vi "calc T.vi"(7 "DAQ state cluster in in":T1 {"T cont"."utility"."therm volt" format="%_6g"; "T cont"."T status"."Temp" format="%_6g"}) -> (8 "DAQ state cluster out":T1 {"T cont"."utility"."therm volt" format="%_6g"; "T cont"."T status"."Temp" format="%_6g"})   [LabVIEW 2019]
doc: "This subVI is a component of the meas T state of the DAQ state machine in the thermistor experiment.\n\nThis subVI calculates the current time and the thermistor temperature from the raw voltage measurement.\n\nPaul K Dixon\nP3600\nCSUSB Physics"
uses:
  typedefs/DAQ T state cluster.ctl
  typedefs/DAQ T state enum.ctl
  typedefs/temp cont cluster.ctl
  typedefs/temp exec cluster.ctl
  typedefs/temp mode enum.ctl
  typedefs/temp indicator.ctl
  typedefs/temp cont utility.ctl
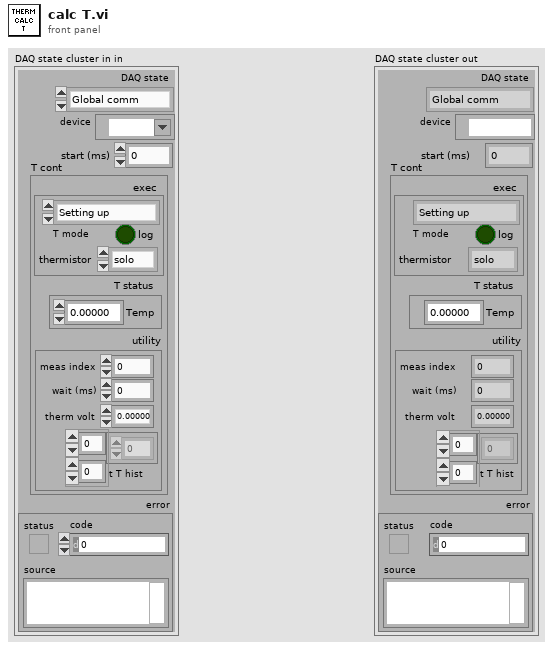
[diagram p1: front panel]
types:
  T1 = typedef "DAQ T state cluster.ctl" = cluster{"DAQ state":T2, "device":tag, "start (ms)":i32, "error":errorcluster, "T cont":T3}
  T2 = typedef "DAQ T state enum.ctl" = enum16{"Global comm", "Meas T ", "Wait", "Exit"}
  T3 = typedef "temp cont cluster.ctl" = cluster{"exec":T4, "T status":T6, "utility":T7}
  T4 = typedef "temp exec cluster.ctl" = cluster{"T mode":T5, "log":bool, "thermistor":enum16{"solo", "bug"}}
  T5 = typedef "temp mode enum.ctl" = enum16{"Setting up", "Listening to exec", "Exit"}
  T6 = typedef "temp indicator.ctl" = cluster{"Temp":dbl}
  T7 = typedef "temp cont utility.ctl" = cluster{"meas index":i32, "wait (ms)":i32, "therm volt":dbl, "t T hist":dbl[][]}
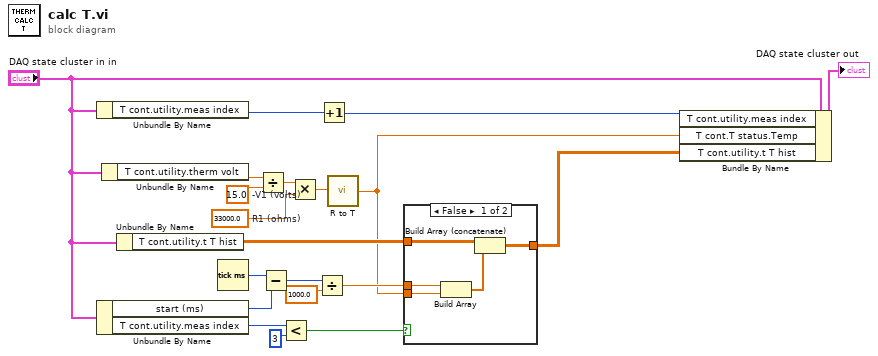
[diagram p0: block diagram]
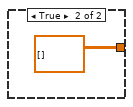
[diagram p2: hidden frame]
diagram:
  w18 = 15.0  # -V1 (volts)
  w16 = 33000.0  # R1 (ohms)
  n1 = Unbundle By Name("DAQ state cluster in in") -> ("T cont.utility.meas index"=w6:i32)
  n2 = Unbundle By Name("DAQ state cluster in in") -> ("start (ms)"=w12:i32, "T cont.utility.meas index"=w4:i32)
  n3 = Unbundle By Name("DAQ state cluster in in") -> ("T cont.utility.therm volt"=w19:dbl)
  n4 = Unbundle By Name("DAQ state cluster in in") -> ("T cont.utility.t T hist"=w14:dbl[][])
  n5 = Tick Count (ms)() -> (millisecond timer value=w13:u32)
  n6 = Divide(x=w19, y=w18) -> (x/y=w17:dbl)
  n7 = Subtract(x=w13, y=w12) -> (x-y=w11:u32)
  n8 = Less?(x=w4, y=3) -> (x < y?=w2:bool)
  n9 = Multiply(x=w17, y=w16) -> (x*y=w15:dbl)
  n10 = Divide(x=w11, y=1000.0) -> (x/y=w8:dbl)
  n11 = Increment(x=w6) -> (x+1=w5:i32)
  n12 = call "R to T.vi"("Resistance (Ohm)"=w15) -> ("Temp (deg C)"=w7:dbl)  [unwired: 13 in, 1 out]
  n13 = case shown="False" w2 {
    tunnel: w14 -> [w25 _]
    tunnel: w8 -> [w24 _]
    tunnel: w7 -> [w23 _]
    tunnel: [w21 dbl[][] []] -> w1
    frame False {
      n14 = Build Array(w24, w23) -> (w22:dbl[])
      n15 = Build Array (concatenate)(w25, w22) -> (w21:dbl[][])
    }
    frame True {
    }
  }
  n16 = Bundle By Name(cluster="DAQ state cluster in in", "T cont.utility.meas index"=w5, "T cont.T status.Temp"=w7, "T cont.utility.t T hist"=w1) -> (→"DAQ state cluster out":T1)
